vi "Intialise or refresh queue.vi"(2 "When did you stick it in?":dbl, 3 "Cell Settings Array":T2(array[cluster])=[{"Measure?"=TRUE, "Area (cm^2)"=0.0, "Cell Label"="", "Cell Description"="", "Time between scans (s)"=0.0, "Cell Position"=1, "Scan settings in queue"=0, "Sample holder"=4.0}, {"Measure?"=TRUE, "Area (cm^2)"=0.0, "Cell Label"="", "Cell Description"="", "Time between scans (s)"=0.0, "Cell Position"=2, "Scan settings in queue"=0, "Sample holder"=4.0}, {"Measure?"=TRUE, "Area (cm^2)"=0.0, "Cell Label"="", "Cell Description"="", "Time between scans (s)"=0.0, "Cell Position"=3, "Scan settings in queue"=0, "Sample holder"=4.0}, {"Measure?"=TRUE, "Area (cm^2)"=0.0, "Cell Label"="", "Cell Description"="", "Time between scans (s)"=0.0, "Cell Position"=4, "Scan settings in queue"=0, "Sample holder"=4.0}, {"Measure?"=TRUE, "Area (cm^2)"=0.0, "Cell Label"="", "Cell Description"="", "Time between scans (s)"=0.0, "Cell Position"=5, "Scan settings in queue"=0, "Sample holder"=4.0}, {"Measure?"=TRUE, "Area (cm^2)"=0.0, "Cell Label"="", "Cell Description"="", "Time between scans (s)"=0.0, "Cell Position"=6, "Scan settings in queue"=0, "Sample holder"=4.0}, {"Measure?"=TRUE, "Area (cm^2)"=0.0, "Cell Label"="", "Cell Description"="", "Time between scans (s)"=0.0, "Cell Position"=7, "Scan settings in queue"=0, "Sample holder"=4.0}, {"Measure?"=TRUE, "Area (cm^2)"=0.0, "Cell Label"="", "Cell Description"="", "Time between scans (s)"=0.0, "Cell Position"=8, "Scan settings in queue"=0, "Sample holder"=4.0}, {"Measure?"=TRUE, "Area (cm^2)"=0.0, "Cell Label"="", "Cell Description"="", "Time between scans (s)"=0.0, "Cell Position"=9, "Scan settings in queue"=0, "Sample holder"=4.0}, {"Measure?"=TRUE, "Area (cm^2)"=0.0, "Cell Label"="", "Cell Description"="", "Time between scans (s)"=0.0, "Cell Position"=10, "Scan settings in queue"=0, "Sample holder"=4.0}, {"Measure?"=TRUE, "Area (cm^2)"=0.0, "Cell Label"="", "Cell Description"="", "Time between scans (s)"=0.0, "Cell Position"=11, "Scan settings in queue"=0, "Sample holder"=4.0}, {"Measure?"=TRUE, "Area (cm^2)"=0.0, "Cell Label"="", "Cell Description"="", "Time between scans (s)"=0.0, "Cell Position"=12, "Scan settings in queue"=0, "Sample holder"=4.0}, {"Measure?"=TRUE, "Area (cm^2)"=0.0, "Cell Label"="", "Cell Description"="", "Time between scans (s)"=0.0, "Cell Position"=13, "Scan settings in queue"=0, "Sample holder"=4.0}, {"Measure?"=TRUE, "Area (cm^2)"=0.0, "Cell Label"="", "Cell Description"="", "Time between scans (s)"=0.0, "Cell Position"=14, "Scan settings in queue"=0, "Sample holder"=4.0}, {"Measure?"=TRUE, "Area (cm^2)"=0.0, "Cell Label"="", "Cell Description"="", "Time between scans (s)"=0.0, "Cell Position"=15, "Scan settings in queue"=0, "Sample holder"=4.0}, {"Measure?"=TRUE, "Area (cm^2)"=0.0, "Cell Label"="", "Cell Description"="", "Time between scans (s)"=0.0, "Cell Position"=16, "Scan settings in queue"=0, "Sample holder"=4.0}] {"Scan settings in queue" items=["Regular", "Inverted"]}, 4 "Queue in":T1(array[cluster]) {"Scan settings in queue" items=["Regular", "Inverted"]; "Time of the last scan (s)" format="%<%H:%M:%S>t"; "When did you stick it in?" format="%<%H:%M:%S>t"; "Time to next scan (s)" format="%<%H:%M:%S>t"; "Time in rig (s)" format="%<%H:%M:%S>t"}) -> (0 "Queue out":T1(array[cluster]) {"Scan settings in queue" items=["Regular", "Inverted"]; "Time of the last scan (s)" format="%<%H:%M:%S>t"; "When did you stick it in?" format="%<%H:%M:%S>t"; "Time to next scan (s)" format="%<%H:%M:%S>t"; "Time in rig (s)" format="%<%H:%M:%S>t"})   [LabVIEW 2011]
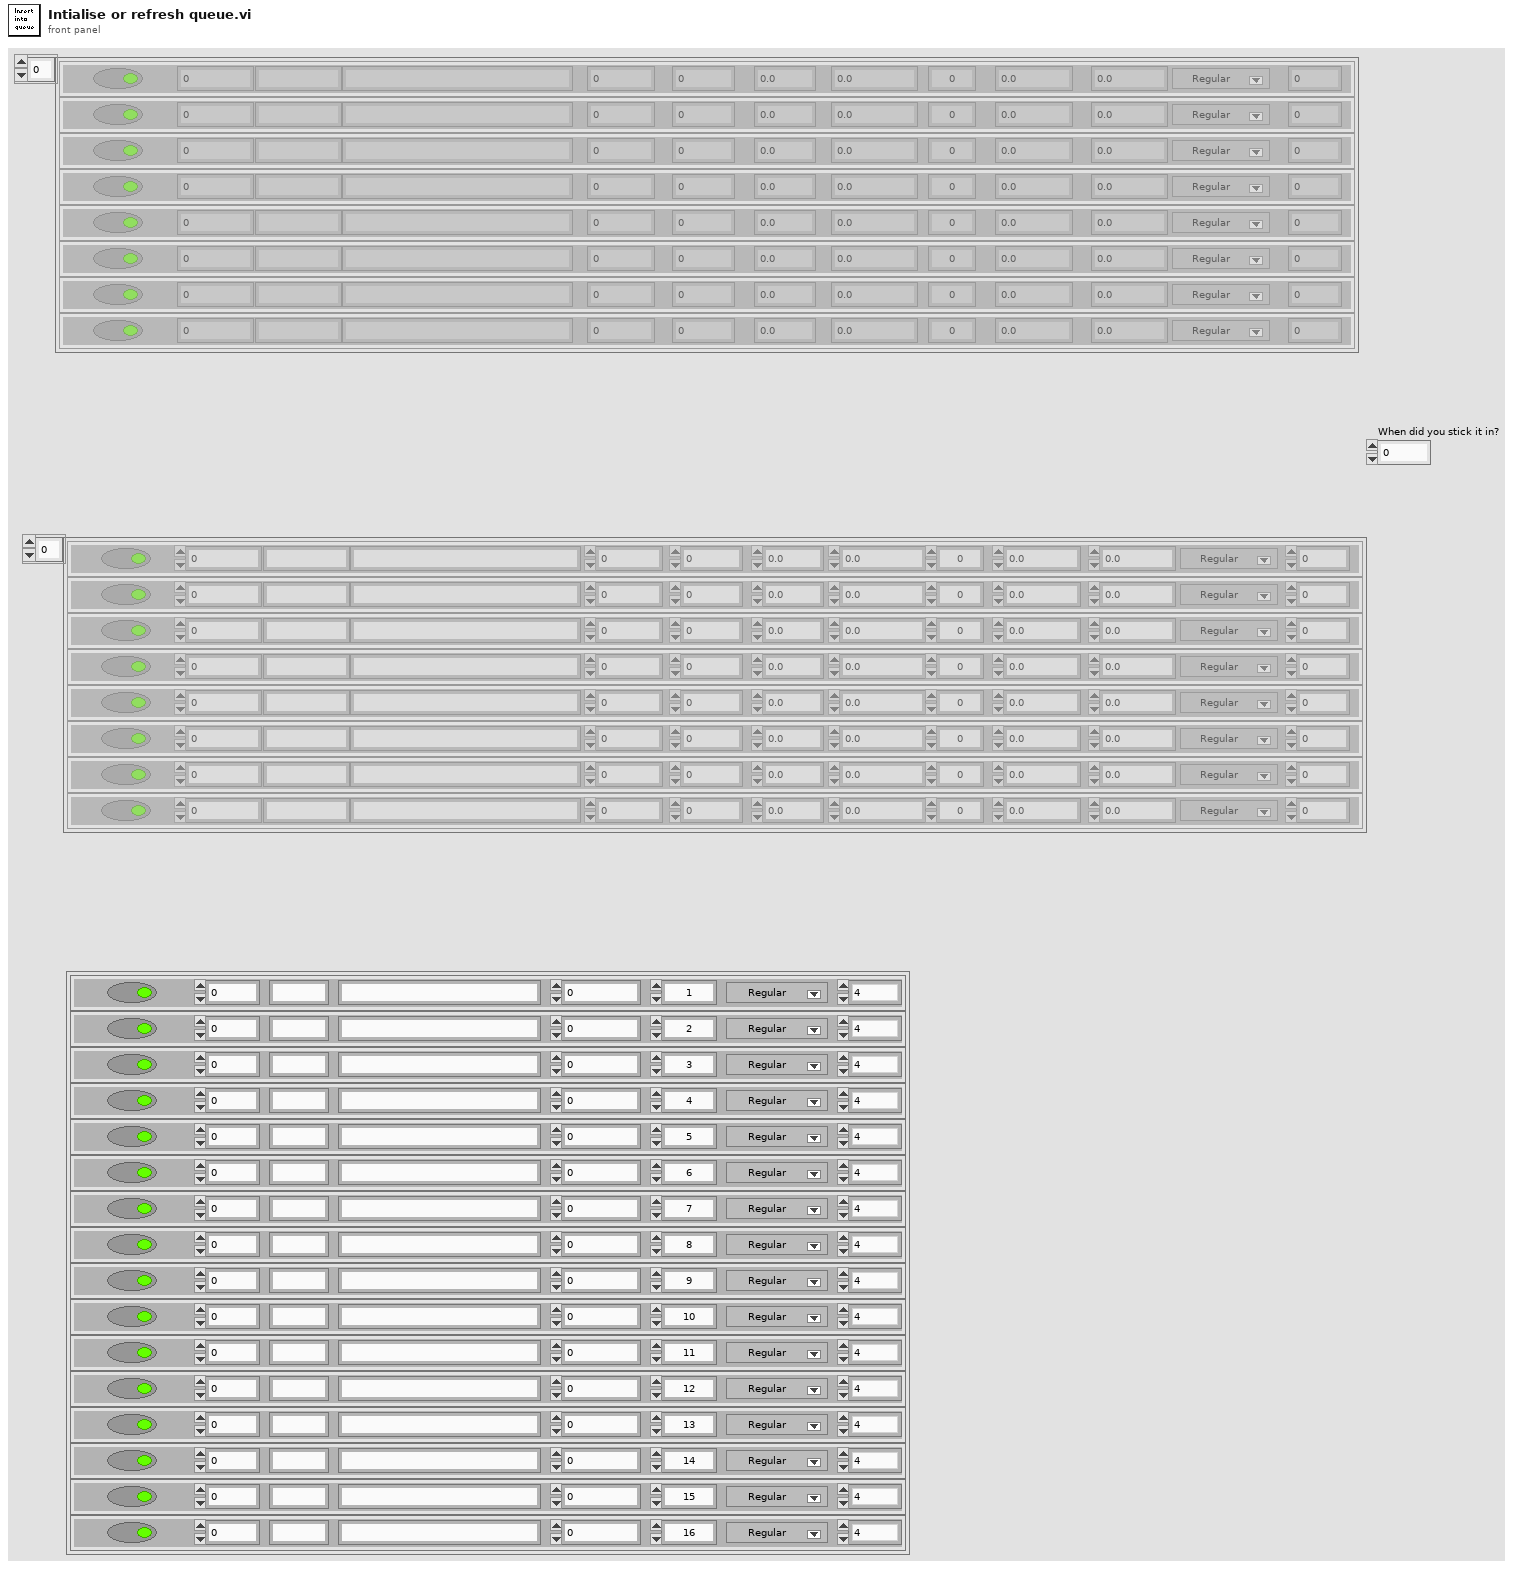
[diagram p1: front panel]
types:
  T1 = cluster{"Measure?":bool, "Area (cm^2)":dbl, "Cell Label":string, "Cell Description":string, "Cell Position":i32, "Time in rig (s)":dbl, "Time to next scan (s)":dbl, "Scan number":dbl, "When did you stick it in?":dbl, "Time between scans (s)":dbl, "Time of the last scan (s)":dbl, "Scan settings in queue":u16, "Sample Holder":dbl}[]
  T2 = cluster{"Measure?":bool, "Area (cm^2)":dbl, "Cell Label":string, "Cell Description":string, "Time between scans (s)":dbl, "Cell Position":i32, "Scan settings in queue":u16, "Sample holder":dbl}[]
  T3 = cluster{"Measure?":bool, "Area (cm^2)":dbl, "Cell Label":string, "Cell Description":string, "Cell Position":i32, "Time in rig (h)":dbl, "Time to next scan (min)":dbl, "Scan number":dbl, "When did you stick it in?":dbl, "Time between scans (min)":dbl, "Time of the last scan(min)":dbl, "Scan settings in queue":u16, "Sample Holder":dbl}[]
  T4 = cluster{"Measure?":bool, "Area (cm^2)":dbl, "Cell Label":string, "Cell Description":string, "Cell Position":i32, "Time in rig (s)":dbl, "Time to next scan (s)":dbl, "Scan number":dbl, "When did you stick it in?":dbl, "Time between scans (s)":dbl, "Time of the last scan (s)":dbl, "Scan settings in queue":u16, "Sample Holder":dbl}
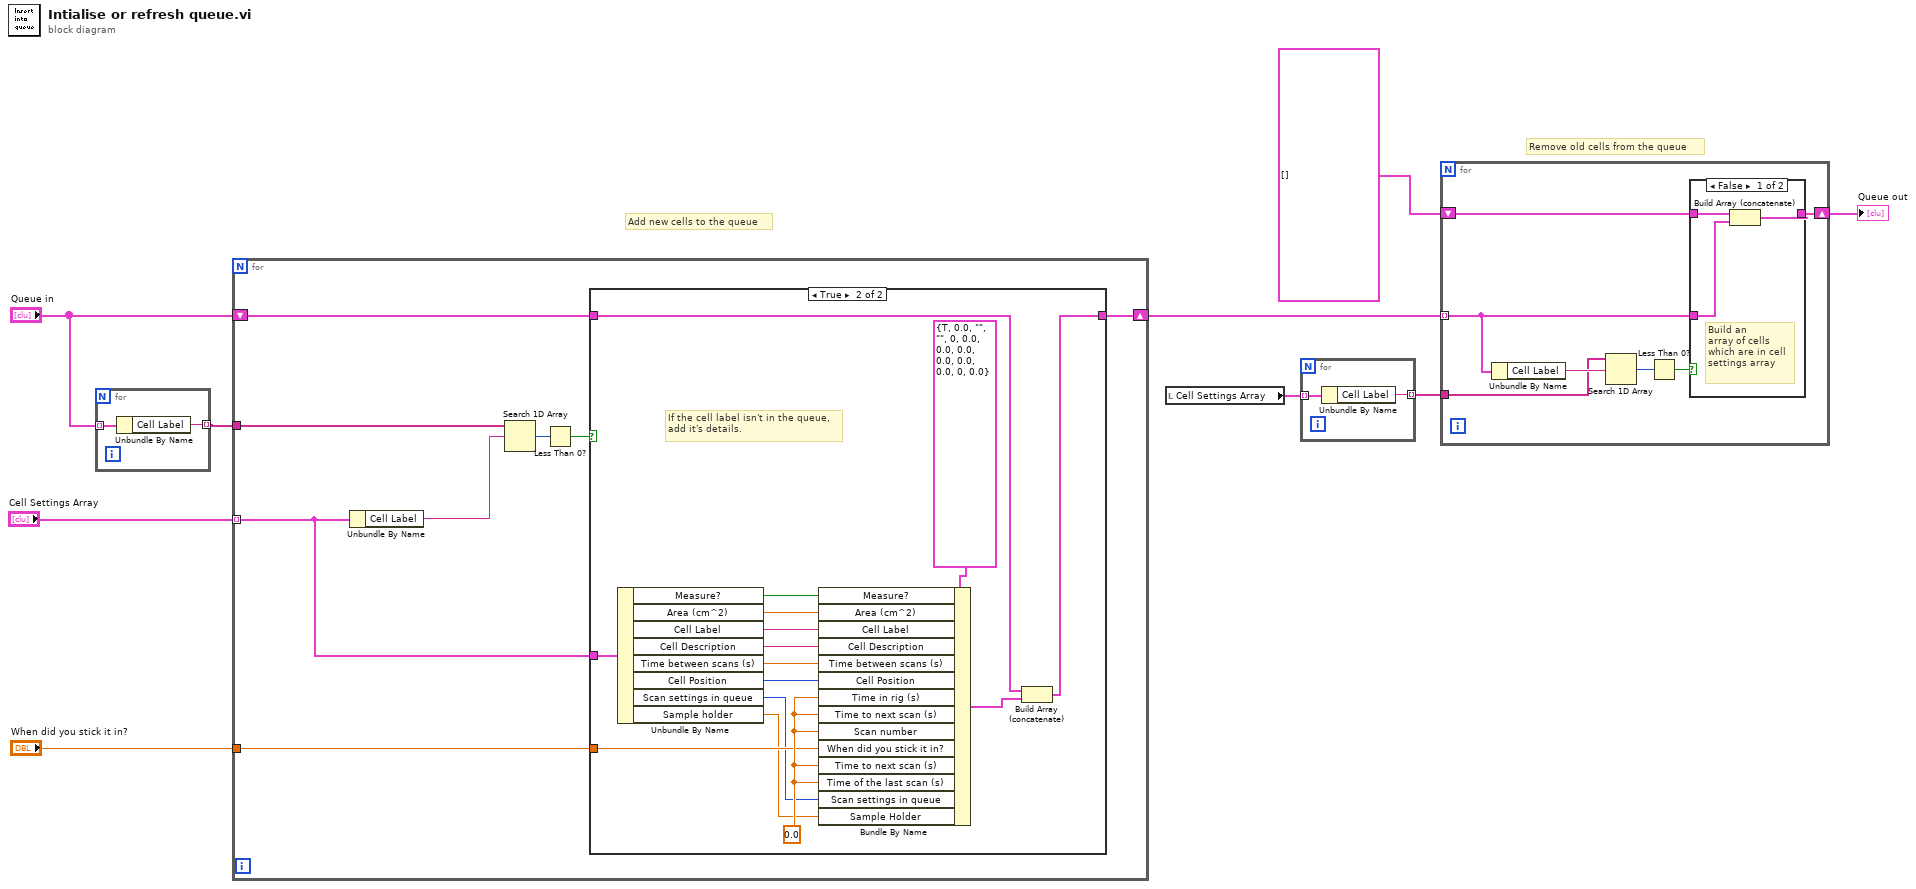
[diagram p0: block diagram]
diagram:
  # "Remove old cells from the queue"
  # "Add new cells to the queue"
  n1 = for {
    tunnel: "Queue in" -> [w11] mode=indexing
    tunnel: [w10] -> w8 mode=indexing
    n2 = Unbundle By Name(w11) -> ("Cell Label"=w10:string)
  }
  n3 = for {
    tunnel: "Cell Settings Array" -> [w14] mode=indexing
    tunnel: "When did you stick it in?" -> [w15]
    tunnel: w8 -> [w17]
    shift-right: [w12] -> w6
    shift-left: "Queue in" -> [w13]
    n4 = Unbundle By Name(w14) -> ("Cell Label"=w19:string)
    n5 = Search 1D Array(1D array=w17, element=w19) -> (index of element=w18:i32)  [unwired: 1 in]
    n6 = Less Than 0?(x=w18) -> (x < 0?=w16:bool)
    n7 = case shown="True" w16 {
      tunnel: w15 -> [_ w33]
      tunnel: w14 -> [_ w32]
      tunnel: w13 -> [w20 w23]
      tunnel: [w20 w22] -> w12
      frame False {
      }
      frame True {
        w35 = 0.0 ("Time of the last scan (min)")
        # "If the cell label isn't in the queue,\nadd it's details."
        n8 = Unbundle By Name(w32) -> ("Measure?"=w31:bool, "Area (cm^2)"=w30:dbl, "Cell Label"=w29:string, "Cell Description"=w28:string, "Time between scans (s)"=w27:dbl, "Cell Position"=w26:i32, "Scan settings in queue"=w25:u16, "Sample holder"=w21:dbl)
        n9 = Bundle By Name(cluster=T4 {"Measure?"=TRUE, "Area (cm^2)"=0.0, "Cell Label"="", "Cell Description"="", "Cell Position"=0, "Time in rig (s)"=0.0, "Time to next scan (s)"=0.0, "Scan number"=0.0, "When did you stick it in?"=0.0, "Time between scans (s)"=0.0, "Time of the last scan (s)"=0.0, "Scan settings in queue"=0, "Sample Holder"=0.0} ("Cluster"), "Measure?"=w31, "Area (cm^2)"=w30, "Cell Label"=w29, "Cell Description"=w28, "Time between scans (s)"=w27, "Cell Position"=w26, "Time in rig (s)"=w35, "Time to next scan (s)"=w35, "Scan number"=w35, "When did you stick it in?"=w33, "Time to next scan (s)"=w35, "Time of the last scan (s)"=w35, "Scan settings in queue"=w25, "Sample Holder"=w21) -> (w24:T4)
        n10 = Build Array (concatenate)(w23, w24) -> (w22:T1)
      }
    }
  }
  n11 = local read "Cell Settings Array"() -> (w3:T2)
  n12 = for {
    tunnel: w3 -> [w37] mode=indexing
    tunnel: [w36] -> w7 mode=indexing
    n13 = Unbundle By Name(w37) -> ("Cell Label"=w36:string)
  }
  n14 = for {
    tunnel: w7 -> [w43]
    tunnel: w6 -> [w39] mode=indexing
    shift-right: [w38] -> w1
    shift-left: T3 [] -> [w41]
    n15 = Unbundle By Name(w39) -> ("Cell Label"=w44:string)
    n16 = Search 1D Array(1D array=w43, element=w44) -> (index of element=w42:i32)  [unwired: 1 in]
    n17 = Less Than 0?(x=w42) -> (x < 0?=w40:bool)
    n18 = case shown="False" w40 {
      tunnel: w41 -> [w47 w48]
      tunnel: w39 -> [w46 _]
      tunnel: [w45 w48] -> w38
      frame False {
        # "Build an\narray of cells\nwhich are in cell\nsettings array"
        n19 = Build Array (concatenate)(w47, w46) -> (w45:T1)
      }
      frame True {
      }
    }
  }
  "Queue out" <- w1
